vi "Kelvinox_Parse_Thermometer_Number_to_Excitation.vi"(1 "Excitation Level":dbl) -> (0 "Excitation String":string)   [LabVIEW 2019]
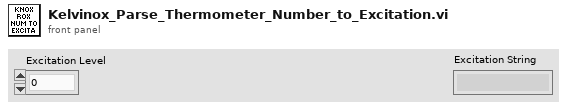
[diagram p1: front panel]
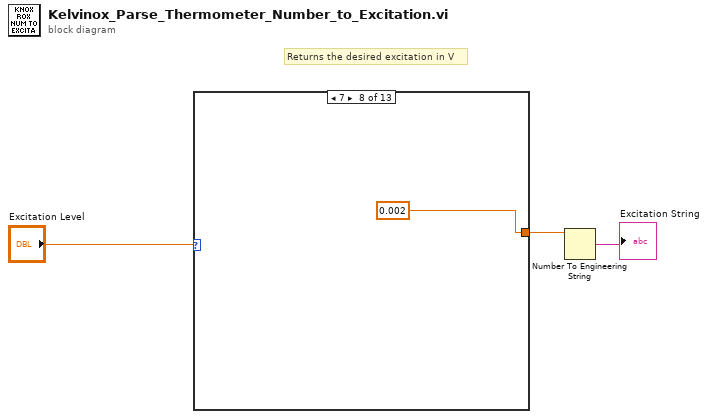
[diagram p0: block diagram]
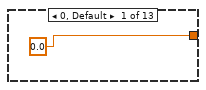
[diagram p2: hidden frame]
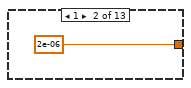
[diagram p3: hidden frame]
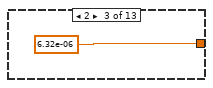
[diagram p4: hidden frame]
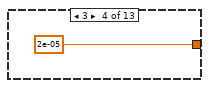
[diagram p5: hidden frame]
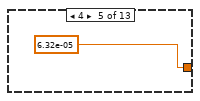
[diagram p6: hidden frame]
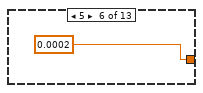
[diagram p7: hidden frame]
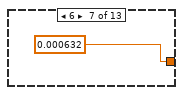
[diagram p8: hidden frame]
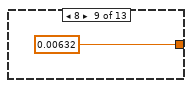
[diagram p9: hidden frame]
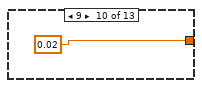
[diagram p10: hidden frame]
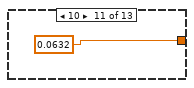
[diagram p11: hidden frame]
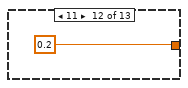
[diagram p12: hidden frame]
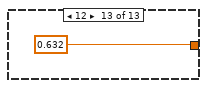
[diagram p13: hidden frame]
diagram:
  # "Returns the desired excitation in V"
  n1 = case shown="7" "Excitation Level" {
    tunnel: [0.0 2e-06 6.32e-06 2e-05 6.32e-05 0.0002 0.000632 0.002 0.00632 0.02 0.0632 0.2 0.632] -> w1
    frame 0, Default {
    }
    frame 1 {
    }
    frame 2 {
    }
    frame 3 {
    }
    frame 4 {
    }
    frame 5 {
    }
    frame 6 {
    }
    frame 7 {
    }
    frame 8 {
    }
    frame 9 {
    }
    frame 10 {
    }
    frame 11 {
    }
    frame 12 {
    }
  }
  n2 = Number To Engineering String(4:w1) -> (0:→"Excitation String":string)  [unwired: 3 in]
